vi "Init Tree and Error Log.vi"(8 "error in (no error)":errorcluster, 11 "Post Analysis in":refnum<class "Post Analysis.lvclass">) -> (0 "error out":errorcluster, 3 "Post Analysis out":refnum<class "Post Analysis.lvclass">)   [LabVIEW 2023, in "Data Analysis.lvlib" / "Post Analysis.lvlib" / "Post Analysis.lvclass"]
uses:
  Post Analysis.lvclass
  Post Analysis.lvclass/Post Analysis.ctl
  HardwareAbstractionLayer_LVOOP/Database/Database.lvclass
panel:
  in  "Test Log(Schema)":string=" edcu_48v_thermal_endurance_test_dv_28_10_2024_19_48_44.error_log" caption="Test Log"
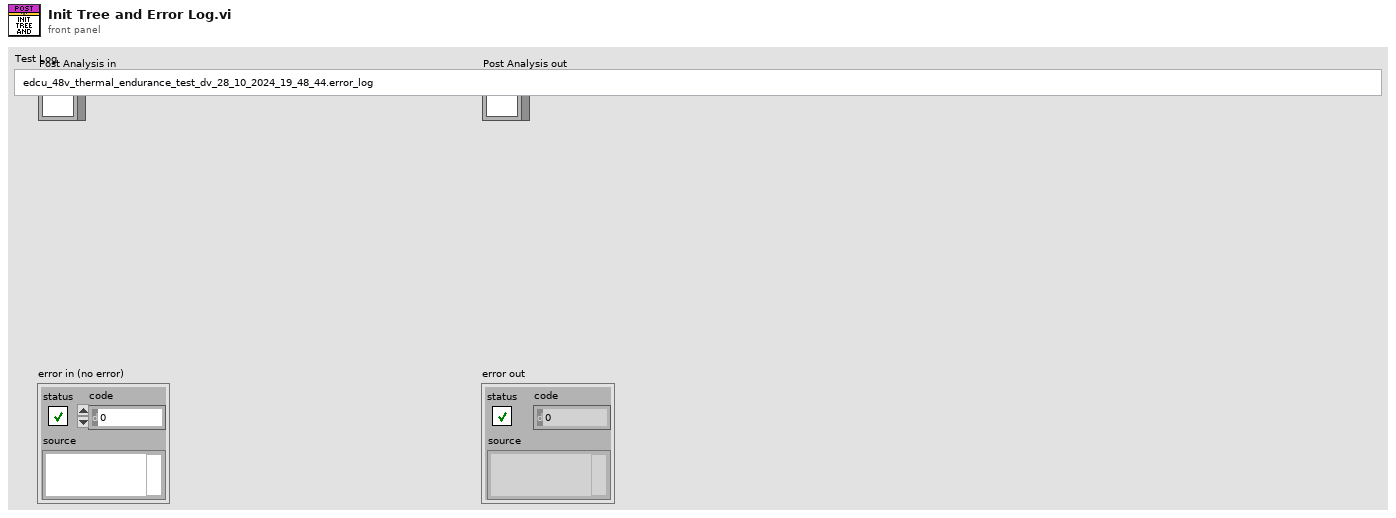
[diagram p1: front panel]
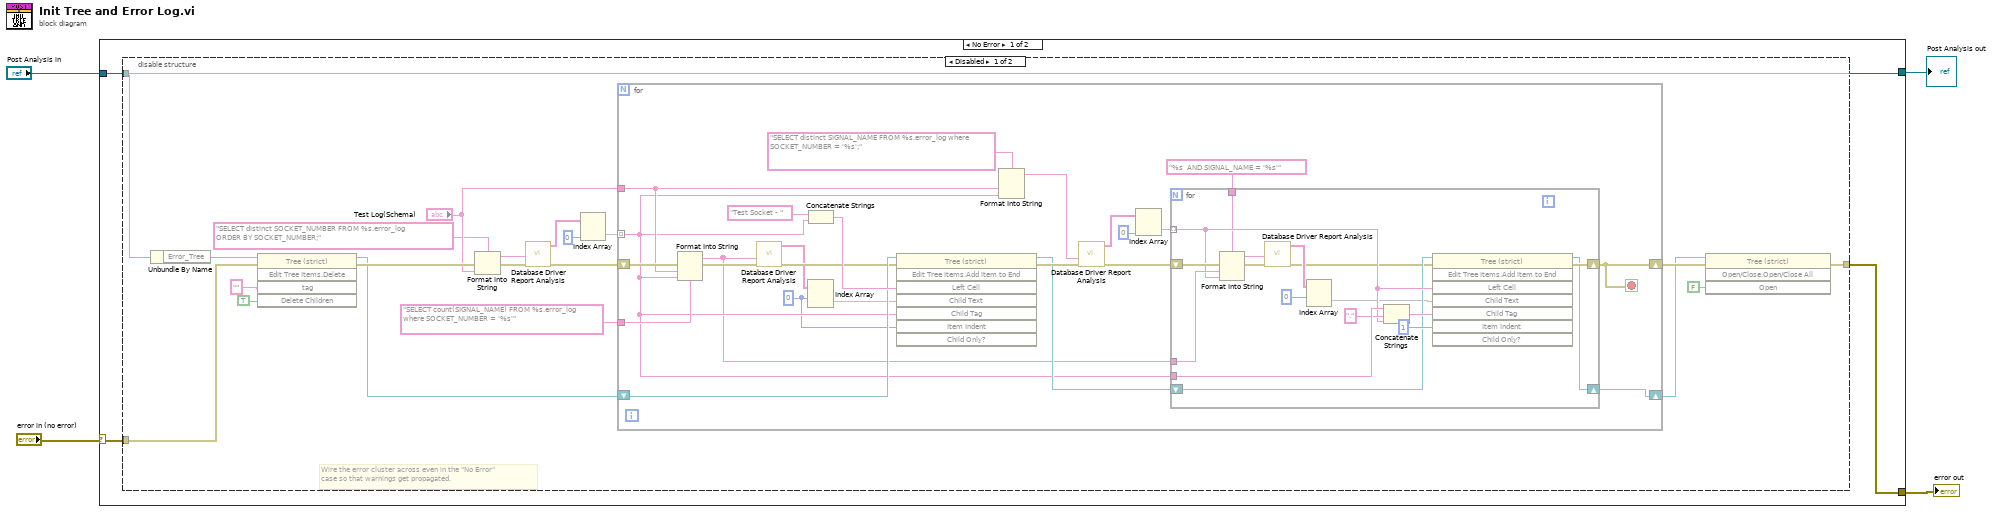
[diagram p0: block diagram]
diagram:
  n1 = case shown="No Error" "error in (no error)" {
    selector: "error in (no error)" -> [w7 w70]
    tunnel: [w6 w70] -> w3
    tunnel: [w5 w69] -> w1
    tunnel: "Post Analysis in" -> [w5 w69]
    frame No Error {
      n2 = disable-structure shown="Disabled" {
        disable-tunnel: w7 -> [w11 _]
        disable-tunnel: [w10 _] -> w6
        disable-tunnel: w5 -> [w9 _]
        frame Disabled {
          # "Wire the error cluster across even in the \"No Error\"\ncase so that warnings get propagated."
          n3 = Unbundle By Name(w9) -> ("Error_Tree"=w8:refnum<vi>)
          n4 = invoke on="Invoke Node" class="Tree (strict)" method="Edit Tree Items.Delete"(reference=w8, error in=w11, "tag"="" ("Tag"), "Delete Children"=TRUE ("Delete Children?")) -> (reference out=w12:refnum<vi>, error out=w25:errorcluster)  [unwired: 1 in, 3 out]
          n5 = Format Into String(format string="SELECT distinct SOCKET_NUMBER FROM %s.error_log ORDER BY SOCKET_NUMBER;" ("SQL query"), error in=w25, "Test Log(Schema)") -> (resulting string=w21:string, error out=w26:errorcluster)  [unwired: 1 in]
          n6 = call "Database Driver Report Analysis.vi"("error in"=w26, "SQL query"=w21) -> ("error out"=w17:errorcluster, "data"=w18:string[][])  [unwired: 6 in, 2 out]
          n7 = Index Array(array=w18, index (col)=0 ("disabled index (col)")) -> (element=w19:string[])  [unwired: 1 in]
          n8 = for {
            tunnel: w19 -> [w33] mode=indexing
            shift-right: [w49] -> w27
            shift-left: w17 -> [w37]
            tunnel: "Test Log(Schema)" -> [w34]
            shift-right: [w39] -> w14
            shift-left: w12 -> [w41]
            tunnel: "SELECT count(SIGNAL_NAME) FROM %s.error_log where SOCKET_NUMBER = '%s'" ("SQL query") -> [w35]
            stop <- w49 stop-if-true
            w30 = 0 ("index (row)")
            n9 = Format Into String(format string=w35, error in=w37, w34, w33) -> (resulting string=w29:string, error out=w36:errorcluster)  [unwired: 1 in]
            n10 = call "Database Driver Report Analysis.vi"("error in"=w36, "SQL query"=w29) -> ("error out"=w38:errorcluster, "data"=w32:string[][])  [unwired: 6 in, 2 out]
            n11 = Index Array(array=w32, index (row)=w30) -> (element=w31:string[])  [unwired: 1 in]
            n12 = Concatenate Strings("Test Socket - " ("element"), w33) -> (w50:string)
            n13 = invoke on="Invoke Node" class="Tree (strict)" method="Edit Tree Items.Add Item to End"(reference=w41, error in=w38, "Left Cell"=w50, "Child Text"=w31, "Child Tag"=w33, "Item Indent"=w30) -> (reference out=w40:refnum<vi>, error out=w48:errorcluster)  [unwired: 2 in, 6 out]
            n14 = Format Into String(format string="SELECT distinct SIGNAL_NAME FROM %s.error_log where SOCKET_NUMBER = '%s';" ("SQL query"), w34, w33) -> (resulting string=w45:string)  [unwired: 2 in, 1 out]
            n15 = call "Database Driver Report Analysis.vi"("error in"=w48, "SQL query"=w45) -> ("error out"=w47:errorcluster, "data"=w43:string[][])  [unwired: 6 in, 2 out]
            n16 = Index Array(array=w43, index (col)=0 ("disabled index (col)")) -> (element=w42:string[])  [unwired: 1 in]
            n17 = for {
              shift-right: [w68] -> w49
              shift-left: w47 -> [w62]
              tunnel: w42 -> [w60] mode=indexing
              tunnel: w33 -> [w66]
              shift-right: [w63] -> w39
              shift-left: w40 -> [w58]
              tunnel: w29 -> [w61]
              tunnel: "%s  AND SIGNAL_NAME = '%s'" ("format string") -> [w59]
              n18 = Format Into String(format string=w59, error in=w62, w61, w60) -> (resulting string=w52:string, error out=w55:errorcluster)  [unwired: 1 in]
              n19 = call "Database Driver Report Analysis.vi"("error in"=w55, "SQL query"=w52) -> ("error out"=w54:errorcluster, "data"=w57:string[][])  [unwired: 6 in, 2 out]
              n20 = Index Array(array=w57, index (row)=0) -> (element=w53:string[])  [unwired: 1 in]
              n21 = Concatenate Strings(w66, "." ("string"), w60) -> (w64:string)
              n22 = invoke on="Invoke Node" class="Tree (strict)" method="Edit Tree Items.Add Item to End"(reference=w58, error in=w54, "Left Cell"=w60, "Child Text"=w53, "Child Tag"=w64, "Item Indent"=1 ("New Item Indentation")) -> (reference out=w63:refnum<vi>, error out=w68:errorcluster)  [unwired: 2 in, 6 out]
            }
          }
          n23 = invoke on="Invoke Node" class="Tree (strict)" method="Open/Close.Open/Close All"(reference=w14, error in=w27, "Open"=FALSE ("Open?")) -> (error out=w10:errorcluster)  [unwired: 1 in, 3 out]
        }
        frame Enabled {
        }
      }
    }
    frame Error {
    }
  }
  "error out" <- w3
  "Post Analysis out" <- w1
